vi "tester.vi"() -> ()   [LabVIEW 2014, in "lvbuildsecurity.lvlib"]
uses:
  lvbuildsecurity.lvlib
  <vilib>/Wiresmith Technology/LabVIEW CLI/CLI Class/CLI.lvclass
panel:
  out "appended path":path
  out "error out":errorcluster
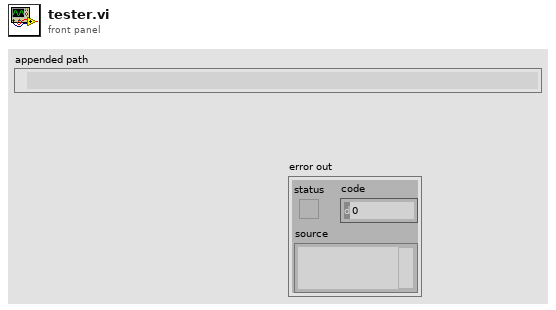
[diagram p1: front panel]
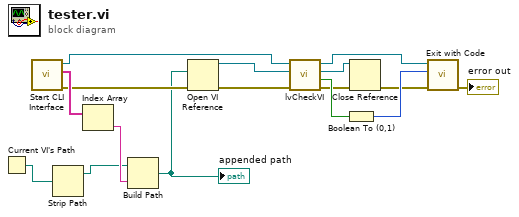
[diagram p0: block diagram]
diagram:
  n1 = Current VI's Path() -> (path=w9:path)
  n2 = call <vilib>:"Start CLI Interface.vi"() -> ("error out"=w7:errorcluster, "Custom Parameters"=w16:string[], "CLI out"=w14:refnum<class "CLI.lvclass">)  [unwired: 9 in]
  n3 = Strip Path(path=w9) -> (stripped path=w8:path)  [unwired: 1 out]
  n4 = Index Array(array=w16) -> (element=w15:string)  [unwired: 1 in]
  n5 = Build Path(base path=w8, name or relative path=w15) -> (appended path=w6:path)
  "appended path" <- w6
  n6 = Open VI Reference(vi path=w6, error in (no error)=w7) -> (vi reference=w5:refnum<vi>, error out=w4:errorcluster)  [unwired: 4 in]
  n7 = call "lvCheckVI.vi"("error in (no error)"=w4, "VI Refnum"=w5, "CLI"=w14) -> ("error out"=w3:errorcluster, "Reject?"=w12:bool, "dup VI Refnum"=w2:refnum<vi>, "CLI out"=w13:refnum<class "CLI.lvclass">)  [unwired: 5 in]
  n8 = Boolean To (0,1)(Boolean=w12) -> (0, 1=w11:i16)
  n9 = Close Reference(reference=w2, error in (no error)=w3) -> (error out=w1:errorcluster)
  n10 = call <vilib>:"Exit with Code.vi"("error in (no error)"=w1, "Exit Code (0)"=w11, "CLI in"=w13) -> ("error out"=→"error out":errorcluster)  [unwired: 8 in]
